vi "Create.vi"(8 "Error In":errorcluster, 11 "Session":refnum<class "Session.lvclass">) -> (0 "Error Out":errorcluster, 3 "Known Hosts":refnum<class "KnownHosts.lvclass">)   [LabVIEW 2017, in "Toolkit.lvlib" / "KnownHosts.lvclass"]
uses:
  KnownHosts.lvclass
  Session/Session.lvclass
  KnownHosts.lvclass/KnownHosts.ctl
  Toolkit.lvlib
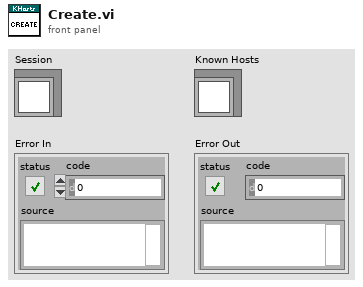
[diagram p1: front panel]
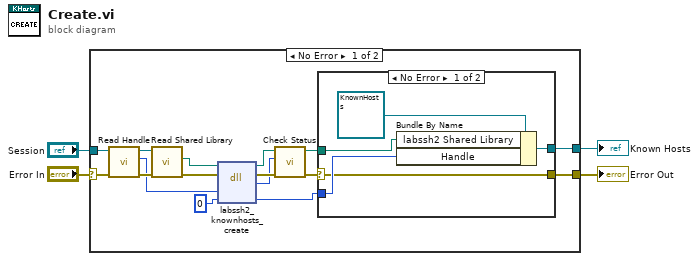
[diagram p0: block diagram]
diagram:
  n1 = case shown="No Error" "Error In" {
    selector: "Error In" -> [w18 w27]
    tunnel: [w5 w27] -> w3
    tunnel: "Session" -> [w19 _]
    tunnel: [w20 _] -> w1
    frame No Error {
      n2 = call "Read Handle.vi"("Error In"=w18, "Session In"=w19) -> ("Erorr Out"=w16:errorcluster, "Handle"=w13:u64, "Session Out"=w17:refnum<class "Session.lvclass">)  [unwired: 7 in]
      n3 = call "Read Shared Library.vi"("Error In"=w16, "Session In"=w17) -> ("Erorr Out"=w15:errorcluster, "labssh2 Shared Library"=w14:path)  [unwired: 7 in, 1 out]
      n4 = dll-call lib="D:/Users/cfield/Code/Field R&D Services/SSH/LabSSH2/LabVIEW/trunk/src/LabSSH2/Private/labssh2.*" fn="labssh2_knownhosts_create"(path in=w14, error in=w15, "session"=w13, "handle"=u64 0) -> (path out=w8:path, error out=w10:errorcluster, "status"=w9:i32, "handle"=w11:u64)  [unwired: 2 in]
      n5 = call "Check Status.vi"("Error In"=w10, "Status"=w9, "labssh2 Shared Library In"=w8) -> ("Error Out"=w7:errorcluster, "labssh2 Shared Library Out"=w6:path)  [unwired: 7 in]
      n6 = case shown="No Error" w7 {
        selector: w7 -> [w21 w26]
        tunnel: [w25 _] -> w20
        tunnel: w11 -> [w23 _]
        tunnel: w6 -> [w22 _]
        tunnel: [w21 w26] -> w5
        frame No Error {
          n7 = Bundle By Name(cluster=refnum<class "KnownHosts.lvclass"> refnum ("LabSSH2.lvlib:KnownHosts.lvclass"), "labssh2 Shared Library"=w22, "Handle"=w23) -> (w25:refnum<class "KnownHosts.lvclass">)
        }
        frame Error {
        }
      }
    }
    frame Error {
    }
  }
  "Error Out" <- w3
  "Known Hosts" <- w1
